vi "process.vi"(8 "error in":errorcluster, 9 "result allocation":T1, 10 "parameters":T1, 11 "ExampleSequencer runtime in":refnum<class "ExampleSequencer runtime.lvclass">) -> (0 "error out":errorcluster, 1 "results":T1, 2 "parameter allocation":T1, 3 "ExampleSequencer runtime out":refnum<class "ExampleSequencer runtime.lvclass">)   [LabVIEW 2017, in "ExampleSequencer runtime.lvclass"]
doc: "Provides an interface for information processing by a module at runtime. While this interface performs no operations, a child should provide an override which may process data in any manner necessary."
uses:
  ExampleSequencer runtime.lvclass
  <vilib>/NI/Tag Bus/table/data table.ctl
  ExampleSequencer runtime.lvclass/ExampleSequencer runtime.ctl
  <vilib>/NI/Tag Bus/table/data table.lvlib
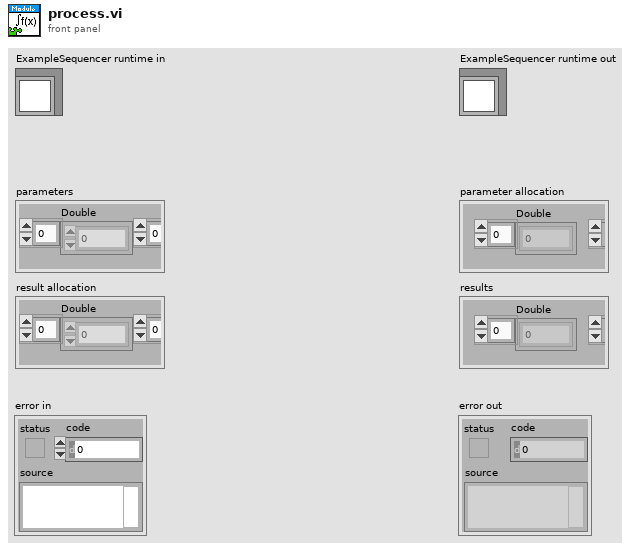
[diagram p1: front panel]
types:
  T1 = typedef "tag bus.lvlib/data table.lvlib/data table.ctl" = cluster{"Double":dbl[], "Single":sgl[], "I64":i64[], "I32":i32[], "I16":i16[], "I8":i8[], "U64":u64[], "U32":u32[], "U16":u16[], "U8":u8[], "Boolean":bool[], "String":string[], "Array of Double":cluster{"DBL Array":dbl[]}[], "Array of Single":cluster{"SGL Array":sgl[]}[], "Array of I64":cluster{"I64 Array":i64[]}[], "Array of I32":cluster{"I32 Array":i32[]}[], "Array of I16":cluster{"I16 Array":i16[]}[], "Array of I8":cluster{"I8 Array":i8[]}[], "Array of U64":cluster{"U64 Array":u64[]}[], "Array of U32":cluster{"U32 Array":u32[]}[], "Array of U16":cluster{"U16 Array":u16[]}[], "Array of U8":cluster{"U8 Array":u8[]}[], "Array of Boolean":cluster{"Boolean Array":bool[]}[], "Array of String":cluster{"String Array":string[]}[]}
  T2 = typedef "ExampleSequencer configuration.lvclass/result data indices.ctl" = cluster{"U16.Controlword":i32, "Array of Double.Parameters":i32}
  T3 = typedef "ExampleSequencer configuration.lvclass/parameter data indices.ctl" = cluster{"U16.Statusword":i32, "Array of Double.Results":i32}
  T4 = typedef "State.ctl" = cluster{"MotionStateMachine_State":T5, "Message_ID":u32, "connection info":T6, "Connected":bool, "Busy":bool, "Current_Parameters":cluster{"Controlword":u16, "Statusword":u16, "Parameters":dbl[], "Results":dbl[]}, "Previous_Parameters":cluster{"P_Controlword":u16, "P_Statusword":u16, "P_Parameters":dbl[], "P_Results":dbl[]}}
  T5 = typedef "WordManipulationLibrary.lvlib/StateMachine.ctl" = enum16{"Start", "Not Ready to Switch On", "Switch On Disabled", "Ready to Switch On", "Switched On", "Operation enable", "Quick Stop Active", "Fault Reaction Active", "Fault"}
  T6 = typedef "NI STM.lvlib/TCP Connection Info.ctl" = cluster{"connection ID":refnum<k5>, "meta data":T7[]}
  T7 = typedef "NI STM.lvlib/MetaDataElement.ctl" = string
  T8 = typedef "ExampleSequencer runtime.lvclass/parameter user data.ctl" = cluster{"Statusword":u16, "Results":dbl[]}
  T9 = cluster{"Controlword":u16, "Statusword":u16, "Parameters":dbl[], "Results":dbl[]}
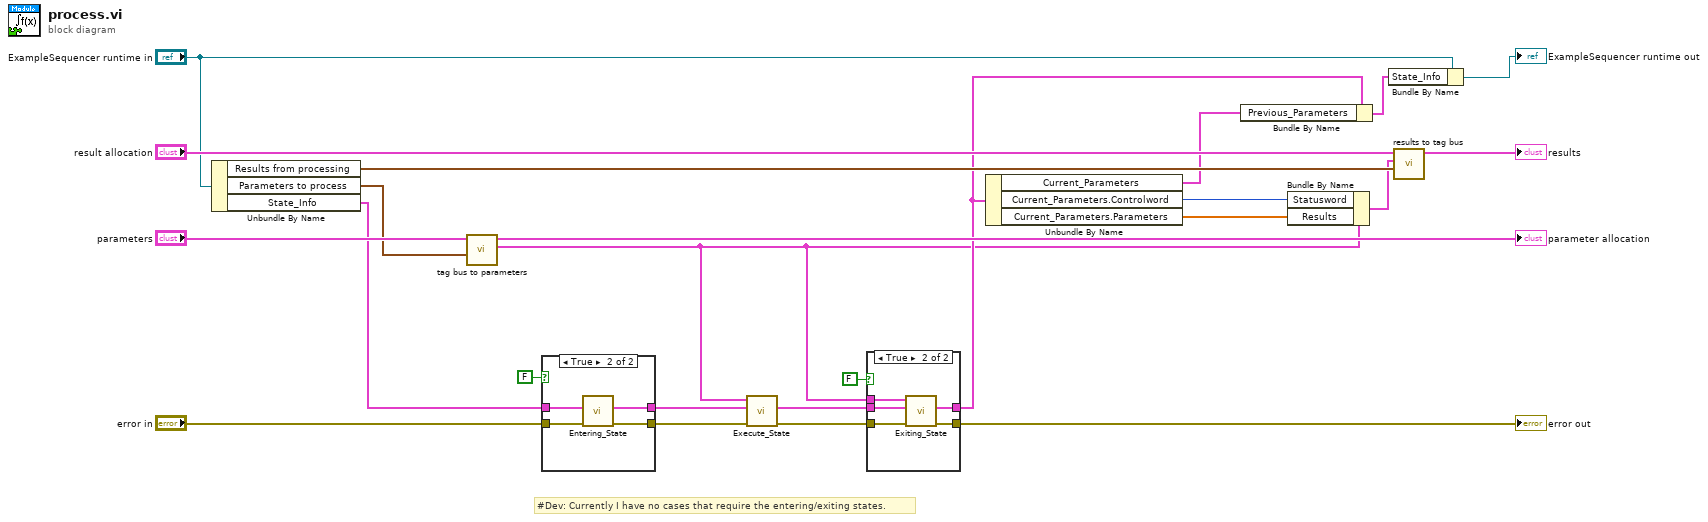
[diagram p0: block diagram]
diagram:
  # "#Dev: Currently I have no cases that require the entering/exiting states."
  n1 = Unbundle By Name("ExampleSequencer runtime in") -> ("Results from processing"=w15:T2, "Parameters to process"=w16:T3, "State_Info"=w14:T4)
  n2 = call "tag bus to parameters.vi"("indices"=w16, "tag bus in"="parameters") -> ("data cluster"=w1:T8, "tag bus out"=→"parameter allocation":T1)  [unwired: 8 in]
  n3 = case shown="True" FALSE {
    tunnel: "error in" -> [w26 w30]
    tunnel: [w26 w29] -> w19
    tunnel: w14 -> [w25 w28]
    tunnel: [w25 w27] -> w13
    frame False {
    }
    frame True {
      n4 = call "Entering_State.vi"("error in"=w30, "State_Info"=w28) -> ("error out"=w29:errorcluster, "State_Info_Out"=w27:T4)  [unwired: 8 in]
    }
  }
  n5 = call "Execute_State.vi"("error in"=w19, "State_Info"=w13, "Parameters to process"=w1) -> ("error out"=w18:errorcluster, "State_Info_Out"=w12:T4)  [unwired: 7 in]
  n6 = case shown="True" FALSE {
    tunnel: w18 -> [w32 w37]
    tunnel: [w32 w36] -> w17
    tunnel: w12 -> [w31 w35]
    tunnel: w1 -> [_ w34]
    tunnel: [w31 w33] -> w4
    frame False {
    }
    frame True {
      n7 = call "Exiting_State.vi"("error in"=w37, "State_Info"=w35, "Parameters to process"=w34) -> ("error out"=w36:errorcluster, "State_Info_Out"=w33:T4)  [unwired: 7 in]
    }
  }
  "error out" <- w17
  n8 = Unbundle By Name(w4) -> ("Current_Parameters"=w2:T9, "Current_Parameters.Controlword"=w7:u16, "Current_Parameters.Parameters"=w6:dbl[])
  n9 = Bundle By Name(cluster=w4, "Previous_Parameters"=w2) -> (w3:T4)
  n10 = Bundle By Name(cluster=w1, "Statusword"=w7, "Results"=w6) -> (w5:T8)
  n11 = Bundle By Name(cluster="ExampleSequencer runtime in", "State_Info"=w3) -> (→"ExampleSequencer runtime out":refnum<class "ExampleSequencer runtime.lvclass">)
  n12 = call "results to tag bus.vi"("indices"=w15, "data cluster"=w5, "tag bus in"="result allocation") -> ("tag bus out"=→"results":T1)  [unwired: 8 in]
